vi "Settings.vi"() -> ()   [LabVIEW 2020, in "Setting Lib.lvlib"]
uses:
  Setting Lib.lvlib
  User Lib.lvlib
panel:
  in  "Calibration":bool
  in  "User":bool
  in  "Close":bool
  in  "General":bool
  # "Settings"
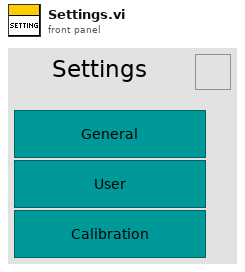
[diagram p1: front panel]
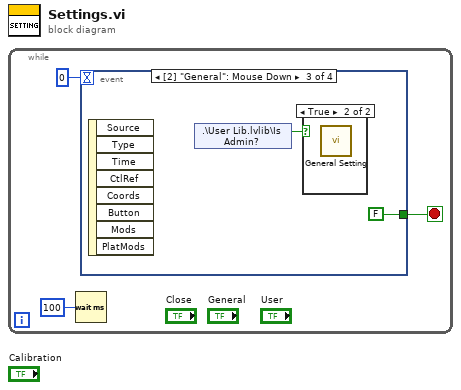
[diagram p0: block diagram]
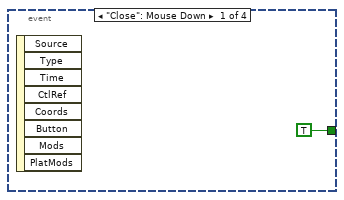
[diagram p2: hidden frame]
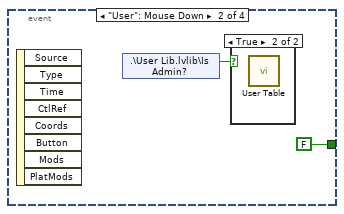
[diagram p3: hidden frame]
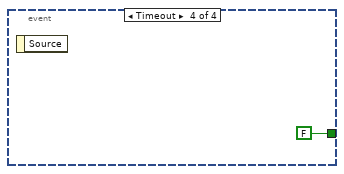
[diagram p6: hidden frame]
diagram:
  n1 = while {
    stop <- w2 stop-if-true
    n2 = Wait (ms)(milliseconds to wait=u32 100) -> ()  [unwired: 1 out]
    n3 = event shown="[2] \"General\": Mouse Down" {
      selector: _ -> [_ _ _ _]
      dyn-events: _ -> [_ _ _ _]
      timeout: 0 -> [_ _ _ _]
      tunnel: [TRUE FALSE FALSE FALSE] -> w2
      event "Close": Mouse Down {
        n4 = event-data() -> ()  [unwired: 1 in, 8 out]
      }
      event "User": Mouse Down {
        n5 = event-data() -> ()  [unwired: 1 in, 8 out]
        n6 = shared-variable ".\\User Lib.lvlib\\Is Admin?"() -> (w6:bool)  [unwired: 1 in, 1 out]
        n7 = case shown="True" w6 {
          frame False {
          }
          frame True {
            n8 = call "User Table.vi"() -> ()  [unwired: 12 in]
          }
        }
      }
      event "General": Mouse Down {
        n9 = event-data() -> ()  [unwired: 1 in, 8 out]
        n10 = shared-variable ".\\User Lib.lvlib\\Is Admin?"() -> (w7:bool)  [unwired: 1 in, 1 out]
        n11 = case shown="True" w7 {
          frame False {
          }
          frame True {
            n12 = call "General Setting.vi"() -> ()  [unwired: 12 in]
          }
        }
      }
      event Timeout {
        n13 = event-data() -> ()  [unwired: 1 in, 1 out]
      }
    }
  }
